vi "Telnet_ping.vi"(4 "Max_trials":i32, 5 "Address":string="192.168.10.152") -> (0 "conn_status":bool)   [LabVIEW 2018]
panel:
  out "ping_resp":string
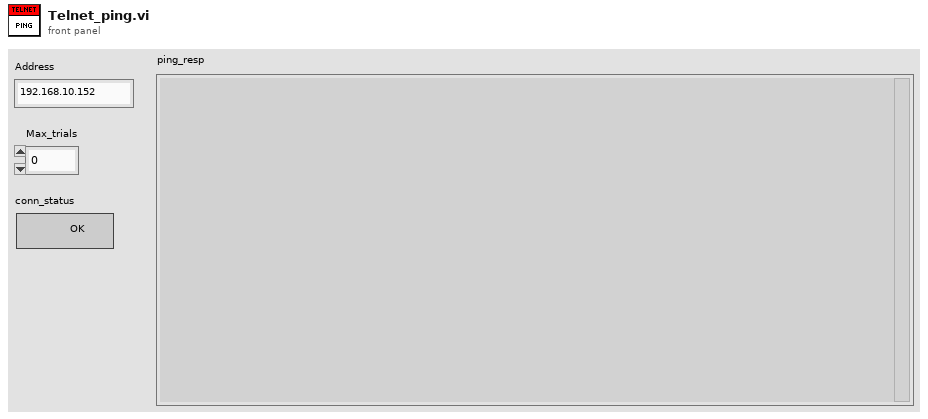
[diagram p1: front panel]
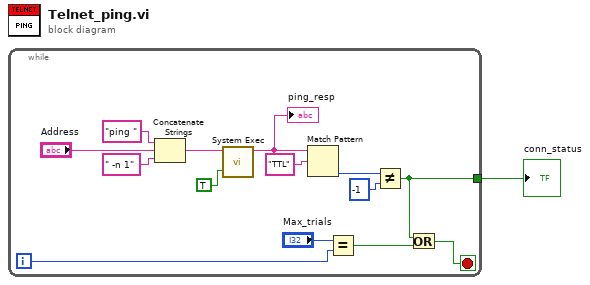
[diagram p0: block diagram]
diagram:
  n1 = while {
    tunnel: [w6] -> w1
    i -> [w5]
    stop <- w7 stop-if-true
    n2 = Concatenate Strings("ping " ("string"), "Address", " -n 1" ("string")) -> (w13:string)
    n3 = call "System Exec.vi"("run minimized? (F)"=TRUE, "command line"=w13) -> ("standard output"=w2:string)  [unwired: 6 in, 3 out]
    "ping_resp" <- w2
    n4 = Match Pattern(string=w2, regular expression="TTL") -> (offset past match=w11:i32)  [unwired: 1 in, 3 out]
    n5 = Equal?(x="Max_trials", y=w5) -> (x = y?=w3:bool)
    n6 = Not Equal?(x=w11, y=-1) -> (x != y?=w6:bool)
    n7 = Or(x=w6, y=w3) -> (x .or. y?=w7:bool)
  }
  "conn_status" <- w1
